vi "Temperature Controller.vi"() -> ()   [LabVIEW 2014]
panel:
  out "Temperature Chart":dynamicdata(graph)
  in  "?":T1(tab)
  in  "Maximum":i32(slide)=35 scale=0.0..60.0
  in  "Minimum":i32(slide)=25 scale=0.0..60.0
  in  "Set Point":dbl(slide)=50.0 scale=0.0..60.0
  in  "Minimum":i32(knob) scale=0.0..60.0
  in  "Maximum":i32(knob)=60 scale=0.0..60.0
  in  "P":dbl(slide)=0.56 scale=0.0..1.8
  in  "D":dbl(slide)=0.2 scale=0.0..1.0
  in  "I":dbl(slide)=0.5 scale=0.0..1.2
  in  "?":bool
  in  "Fan Control":bool
  in  "Heater Control":bool
  in  "Sample/sec":i32(slide)=30 scale=0.0..100.0
  in  "Temperature":i32(knob)=30 scale=0.0..60.0
  in  "?":bool
  out "Moderate":bool=TRUE
  out "Cold":bool
  out "Hot":bool
  out "Thermometer":dbl(slide)=30.0 scale=0.0..60.0
  # "Temperature Controller"
  # "Automatic"
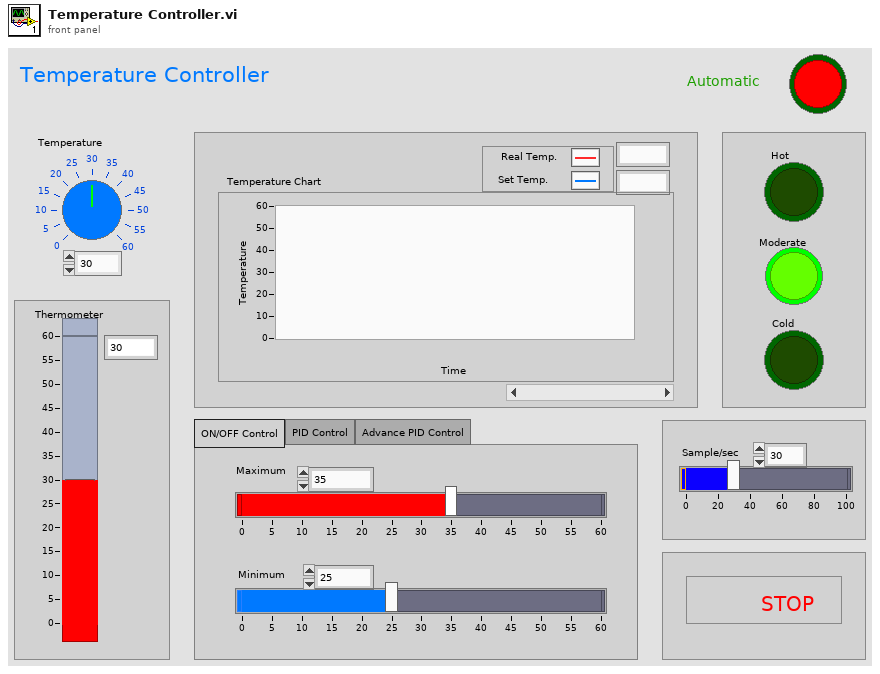
[diagram p1: front panel]
types:
  T1 = enum32{"ON/OFF Control", "PID Control", "Advance PID Control"}
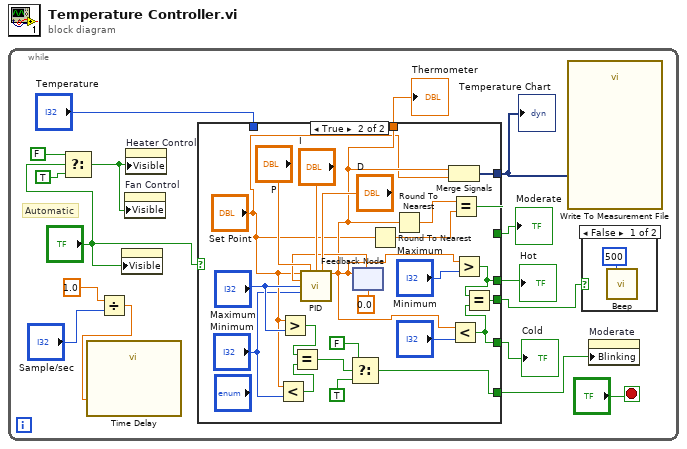
[diagram p0: block diagram]
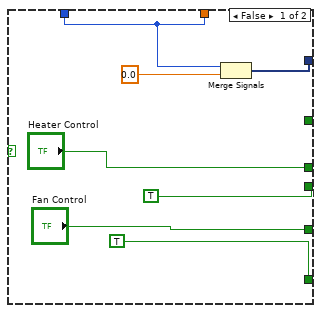
[diagram p2: hidden frame]
diagram:
  n1 = while {
    stop <- "?" stop-if-true
    # "Automatic"
    n2 = Select(t=FALSE, s="?", f=TRUE) -> (s? t:f=w1:bool)
    n3 = Divide(x=1.0, y="Sample/sec") -> (x/y=w9:dbl)
    n4 = call "Time Delay"("Delay Time (s)"=w9) -> ()  [unwired: 10 in, 1 out]
    n5 = property class="TabCtl (strict)"("Visible"="?") -> ()  [unwired: 2 in, 2 out]
    n6 = property on="Fan Control" class="Bool (strict)"("Visible"=w1) -> ()  [unwired: 2 in, 2 out]
    n7 = property on="Heater Control" class="Bool (strict)"("Visible"=w1) -> ()  [unwired: 2 in, 2 out]
    n8 = case shown="True" "?" {
      tunnel: "Temperature" -> [w19 _]
      tunnel: [_ w46] -> w15
      tunnel: ["Heater Control" w45] -> w12
      tunnel: ["Fan Control" w44] -> w14
      tunnel: [TRUE w27] -> w5
      tunnel: [TRUE w43] -> w7
      tunnel: [w19 w34] -> w8
      tunnel: [w17 w33] -> w6
      frame False {
        n9 = Merge Signals(w19, 0.0) -> (w17:dynamicdata)
      }
      frame True {
        n10 = Less?(x="Set Point", y="Minimum") -> (x < y?=w31:bool)
        n11 = Greater?(x="Set Point", y="Maximum") -> (0:w32:bool)
        n12 = Equal?(x=w32, y=w31) -> (x = y?=w26:bool)
        n13 = Select(t=FALSE, s=w26, f=TRUE) -> (s? t:f=w27:bool)
        n14 = feedback #1(0.0 ("output variable")) -> (w38:dbl)
        n15 = call "PID.vi"("sp"="Set Point", "p"="P", "i"="I", "d"="D", "pv"=w38, "maxim"="Maximum", "minim"="Minimum") -> ("output variable"=w34:dbl)  [unwired: 8 in]
        n16 = feedback-in #1(w34) -> ()
        n17 = Round To Nearest(number="Set Point") -> (nearest integer value=w36:dbl)
        n18 = Round To Nearest(number=w34) -> (nearest integer value=w37:dbl)
        n19 = Merge Signals(w34, "Set Point") -> (w33:dynamicdata)
        n20 = Less?(x=w34, y="Minimum") -> (x < y?=w44:bool)
        n21 = Equal?(x=w37, y=w36) -> (x = y?=w46:bool)
        n22 = Greater?(x=w34, y="Maximum") -> (0:w45:bool)
        n23 = Equal?(x=w45, y=w44) -> (x = y?=w43:bool)
      }
    }
    "Thermometer" <- w8
    "Hot" <- w12
    "Cold" <- w14
    "Moderate" <- w15
    "Temperature Chart" <- w6
    n24 = call "Write To Measurement File"("Signals"=w6) -> ()  [unwired: 16 in, 3 out]
    n25 = case shown="False" w7 {
      frame False {
        n26 = call <vilib>:"Beep.vi"("frequency (Hz)"=u32 500) -> ()  [unwired: 11 in]
      }
      frame True {
      }
    }
    n27 = property on="Moderate" class="Bool (strict)"("Blinking"=w5) -> ()  [unwired: 2 in, 2 out]
  }
